vi "SetDigitalOutput.vi"(0 "controller in":refnum<k24>, 5 "axis name":string, 7 "port":i32 min=0 max=2 step=1, 9 "value":i32 min=0 max=255 step=1, 11 "error in (no error)":errorcluster) -> (4 "controller out":refnum<k24>, 15 "error out":errorcluster)   [LabVIEW 2010]
uses:
  c:/aerotech/controller/5.xx.xxx/ensemble/pc/labview/2010/bin/Aerotech.Ensemble.dll
  bin/Aerotech.Ensemble.dll
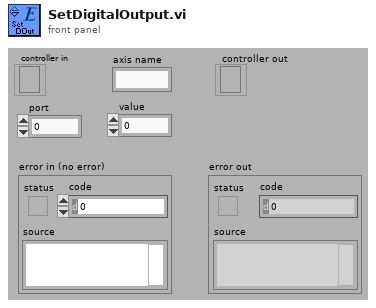
[diagram p1: front panel]
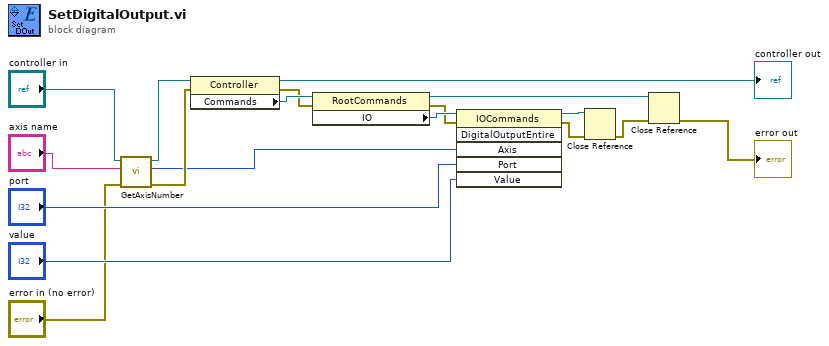
[diagram p0: block diagram]
diagram:
  n1 = call "GetAxisNumber.vi"("error in (no error)"="error in (no error)", "axis name"="axis name", "controller in"="controller in") -> ("error out"=w11:errorcluster, "axis number"=w6:i32, "controller out"=w9:refnum<k24>)  [unwired: 6 in]
  n2 = property class="Controller"(reference=w9, error in=w11) -> (reference out=→"controller out":refnum<k24>, error out=w16:errorcluster, "Commands"=w17:refnum<k24>)
  n3 = property class="RootCommands"(reference=w17, error in=w16) -> (reference out=w1:refnum<k24>, error out=w14:errorcluster, "IO"=w15:refnum<k24>)
  n4 = invoke class="IOCommands" method="DigitalOutputEntire"(reference=w15, error in=w14, "Axis"=w6, "Port"="port", "Value"="value") -> (reference out=w2:refnum<k24>, error out=w3:errorcluster)  [unwired: 1 in, 4 out]
  n5 = Close Reference(reference=w2, error in (no error)=w3) -> (error out=w5:errorcluster)
  n6 = Close Reference(reference=w1, error in (no error)=w5) -> (error out=→"error out":errorcluster)
